vi "CRYStatistics Editor.vi"() -> ()   [LabVIEW 2013]
uses:
  <vilib>/Utility/miscctls.llb/LVBoundsTypeDef.ctl
  Typedef Control/CRYStatistic cluster.ctl
  CRYProject/CRYProject Editor Global.vi
  CRYWindow/SubVI/CRYMain Sub Window Global.vi
  CRYStepSetup/CRYStepSetup Global.vi
  CRYMainGlobal.vi
panel:
  out "Statistics Bk":T1
  in  "CurLibChange":bool caption="Add Lib"
  out "Load_State":bool
  out "EndFlag":bool
  in  "Add Lib":bool=TRUE
  in  "AddStep":bool
  in  "Board Tab":enum32{"Page 1"}(tab)
  in  "Main Tab":enum32{"Setting", "Help"}(tab)
  in  "Sel_Idx":i16
  out "No.Cur Sel":i32 caption="选择曲线个数"
  in  "Mode":u16(slide)
  in  "Sub2 Tab":enum32{"Page 1"}(tab)
  in  "Result Listbox":i32[](listbox)
  in  "AbsMar_StaDev":bool caption="绝对容限标准差"
  in  "Res sigma":i32 caption="+/- 西格玛"
  in  "Mar_Stan Dev":bool caption="容限标准差"
  in  "Margin Mean":bool caption="容限平均值"
  in  "Overall Yield":bool caption="总合格(%)"
  in  "Individual Lim":bool caption="单结果合格(%)"
  out "Result":bool caption="结果"
  in  "Sub1 Tab":enum32{"Page 1"}(tab)
  in  "Data Listbox":i32[](listbox)
  in  "No.Ranked(BF)":i32=1 caption="排" min=1 step=1
  out "LSL Unit":string
  out "USL Unit":string
  in  "LSL":dbl format="%#.2p"
  in  "USL":dbl format="%#.2p"
  in  "Worst Fit":bool caption="最差适合均值"
  in  "Best Fit":bool caption="最佳适合均值"
  in  "Ppk":bool
  in  "Pp":bool
  in  "Abs Stan Dev":bool caption="绝对标准偏差"
  in  "Data sigma":i32 caption="+/- 西格玛"
  in  "Stan Dev":bool caption="标准偏差"
  in  "Mean":bool caption="平均值"
  in  "Min":bool caption="最小值"
  in  "Max":bool caption="最大值"
  out "Data":bool caption="数据"
  in  "No.Ranked(WF)":i32=1 caption="排" min=1 step=1
  in  "Mode xyz":u16(slide) scale=0.0..2.0
  in  "Work in":u16(slide) caption="Work in:"
  in  "Help":string
  in  "Load...":bool caption="Apply"
  in  "Save As...":bool caption="Apply"
  in  "Revert":bool caption="Apply"
  in  "OK":bool caption="Apply"
  in  "Cancel":bool caption="Apply"
  in  "Hardware In":string
  in  "Calibration In":string
  in  "Channel":i32=1
  out "Set up Out":string
  in  "Set up In":string
  in  "stop":bool
  in  "Load Test":bool=TRUE
  in  "Statistics":T1
  out "VIMiniumBound":T2
  in  "Proper VI No":i32
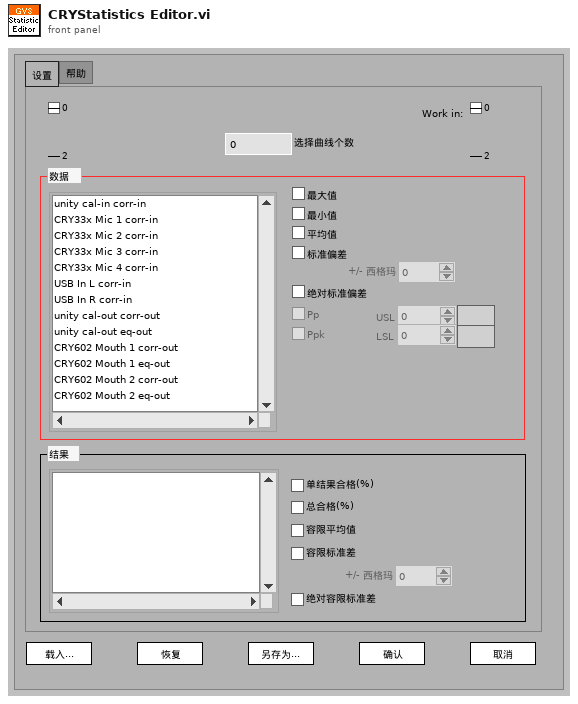
[diagram p1: front panel]
types:
  T1 = typedef "CRYStatistic cluster.ctl" = cluster{"Mode":u16, "No.Ranked(BF)":i32, "No.Ranked(WF)":i32, "Absolute Margin Standard Deviation":bool, "+/- sigma Res":i32, "Margin Standard Deviation":bool, "Margin Mean":bool, "Overall Yield":bool, "Individual Limits Yield":bool, "LSL Unit":string, "USL Unit\n":string, "LSL":dbl, "USL":dbl, "Worst Fit to Average":bool, "Best Fit to Average":bool, "Ppk":bool, "Pp":bool, "Absolute Standard Deviation":bool, "+/- sigma Dat":i32, "Standard Deviation ":bool, "Mean":bool, "Min ":bool, "Max ":bool, "No.of Curves Selected":i32, "Curves":string[], " Results":string[], "Name":string, "Help":string, "Tab Value":enum32{"Setting", "Help"}, "Work in":u16, "Mode xyz":u16}
  T2 = typedef "LVBoundsTypeDef.ctl" = cluster{"Width":u32, "Height":u32}
  T3 = typedef "CRYStep.ctl" = cluster{"No.VI":i32, "Category":string, "StepName":string, "Seq setup flattened":string, "Comment":string, "Steps config.":bool[], "Jump config":i32[], "Start":dbl, "Increment":dbl, "Name":string, "Unit":string, "Y data":u16, "Y prefix":string, "Y dB ref":dbl, "Y unit":string, "Repeat State Array":cluster{"Start":dbl, "Increment":dbl, "Count":i32, "Num":i32}[]}
  T4 = typedef "CRYData Cluster Array.ctl" = T5[]
  T5 = typedef "CRYData Cluster.ctl" = cluster{"Name":string, "Curve":cluster{"x":dbl, "y":dbl, "z":dbl}[], "X data":u16, "Y data":u16, "Z data":u16, "X axis":u16, "Y axis":u16, "Z axis":u16, "X unit":string, "Y unit":string, "Z unit":string, "X dB ref":dbl, "Y dB ref":dbl, "Z dB ref":dbl, "single val":bool, "protected":bool, "display X":bool, "display Y":bool, "display Z":bool, "Test Info":string, "Step No.":i32, "Plot Settings":cluster{"Color":u32, "Interpolation":u8, "Point Style":u8, "Line Style":u8, "Point Color":u32, "Line Width":u8, "Bar Plot Style":u8, "Fill To":i16}, "AutoProtect":bool}
  T6 = typedef "CRYResult Cluster Array.ctl" = T7[]
  T7 = typedef "CRYResult Cluster.ctl" = cluster{"Name":string, "Margin":dbl, "unit":string, "Verdict":bool, "Limit":string, "Max/Min":string, "protected":bool, "Step No.":i32, "Test Info":string, "AutoProtect":bool}
  T8 = enum16{"OK", "Yes", "YesNo", "YesNoCancel", "ReplaceAppend"}
  T9 = enum8{"Enabled", "Disabled", "Disabled and Grayed Out"}
  T10 = cluster{"Load Test":bool, "Add Lib":bool, "OK":bool, "Cancel":bool}
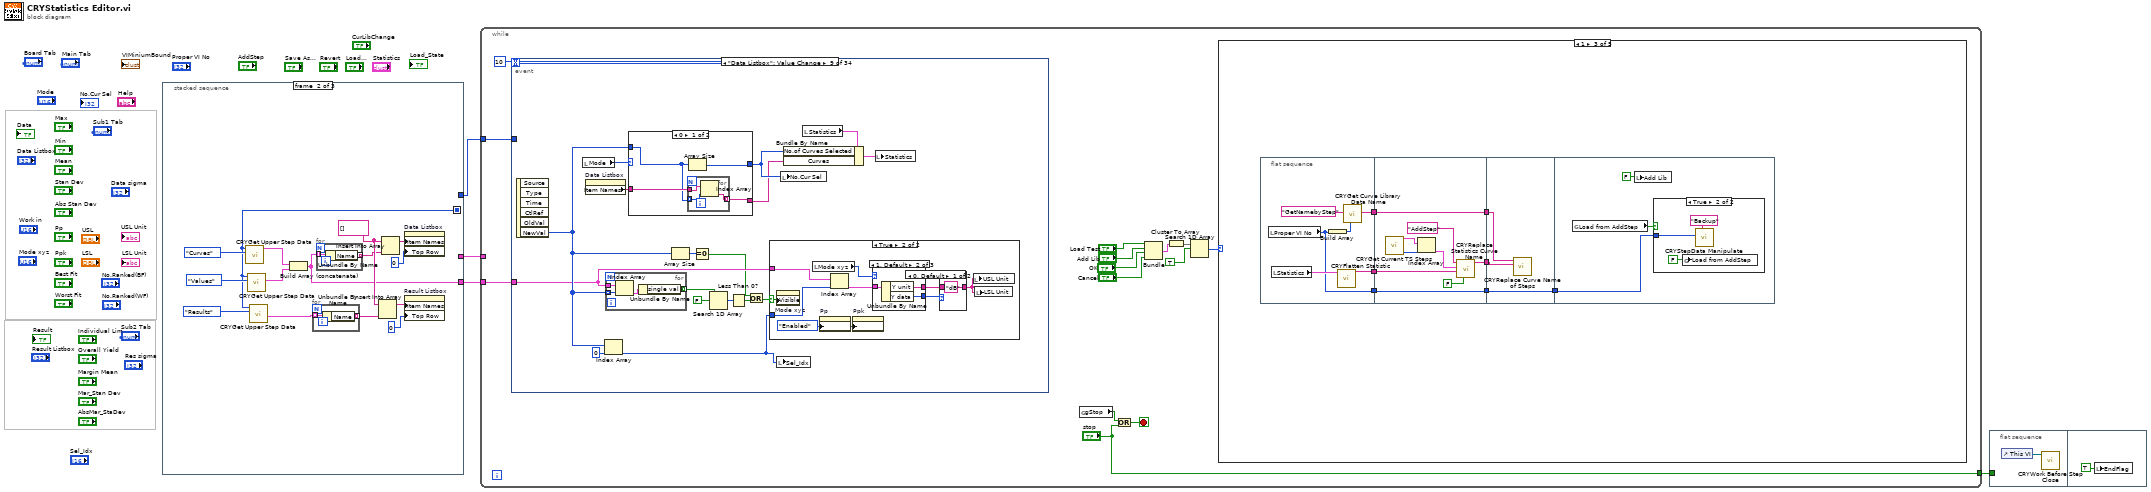
[diagram p0: block diagram]
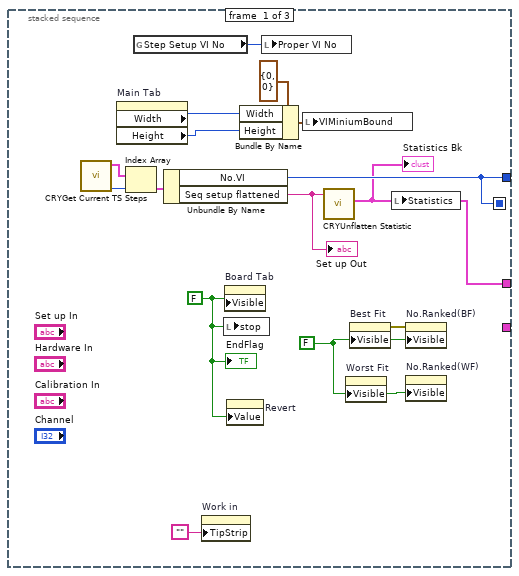
[diagram p2: hidden frame]
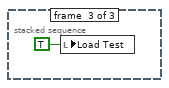
[diagram p3: hidden frame]
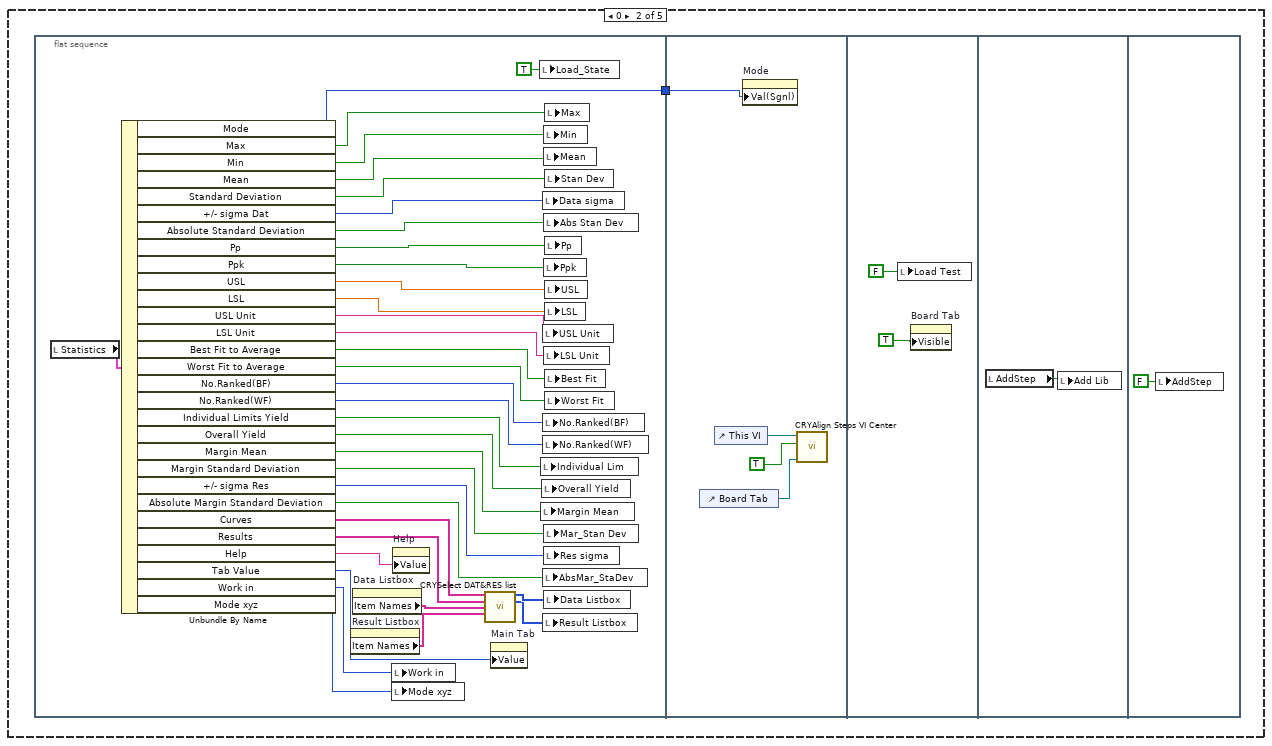
[diagram p5: hidden frame]
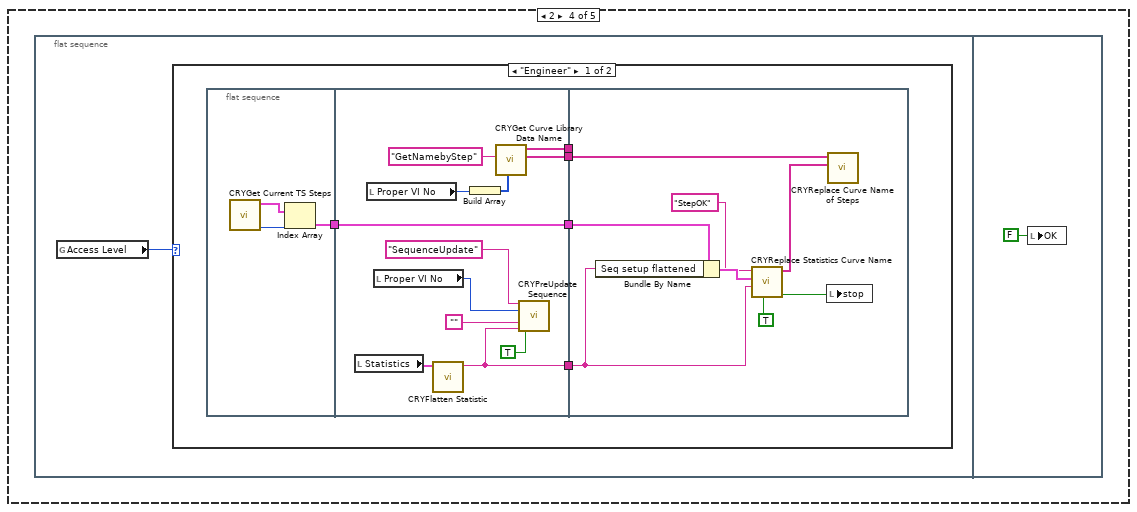
[diagram p7: hidden frame]
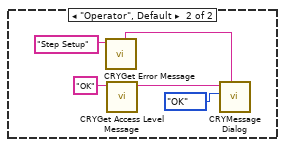
[diagram p8: hidden frame]
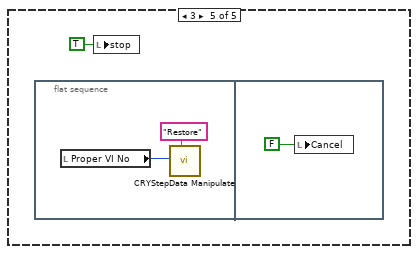
[diagram p9: hidden frame]
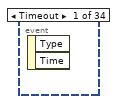
[diagram p10: hidden frame]
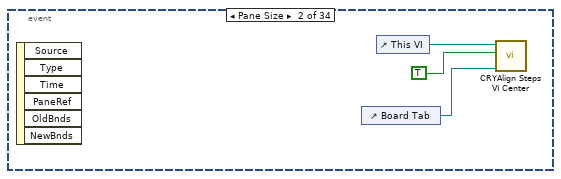
[diagram p11: hidden frame]
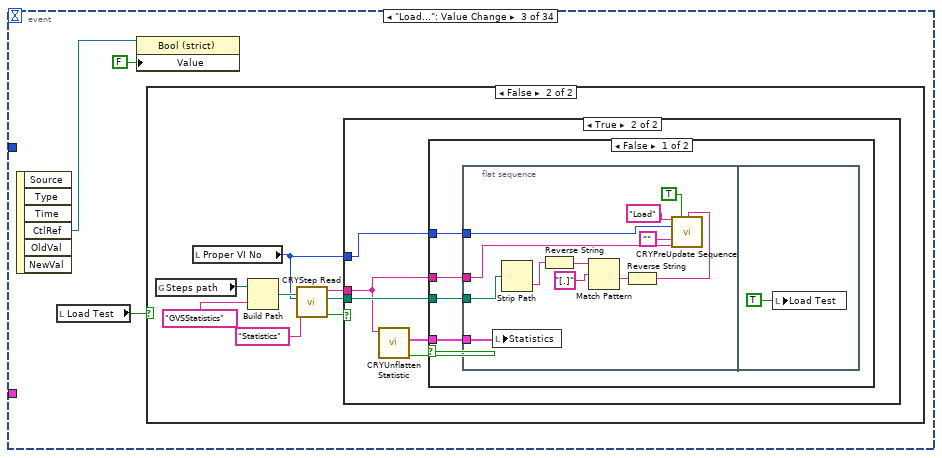
[diagram p12: hidden frame]
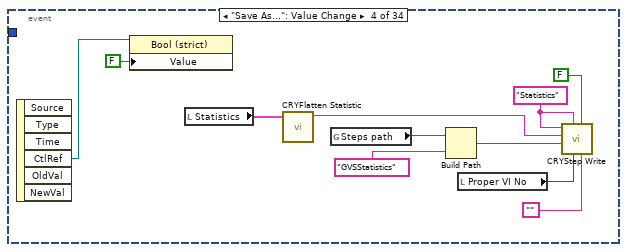
[diagram p16: hidden frame]
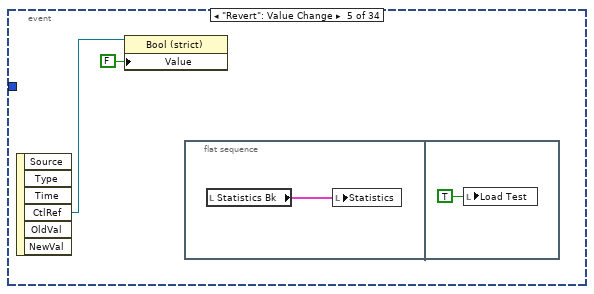
[diagram p17: hidden frame]
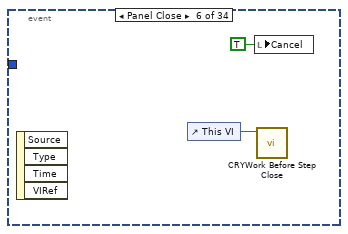
[diagram p18: hidden frame]
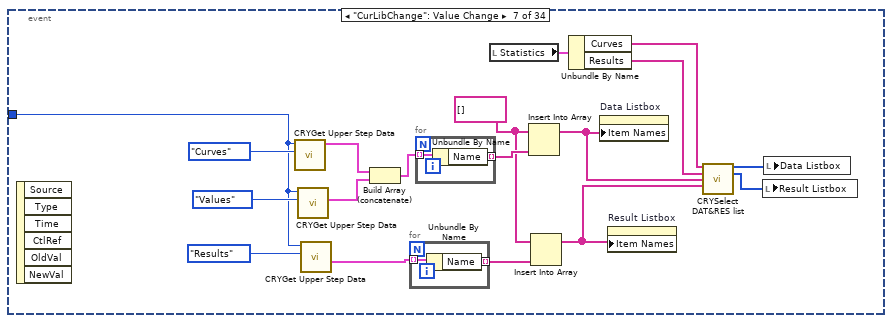
[diagram p19: hidden frame]
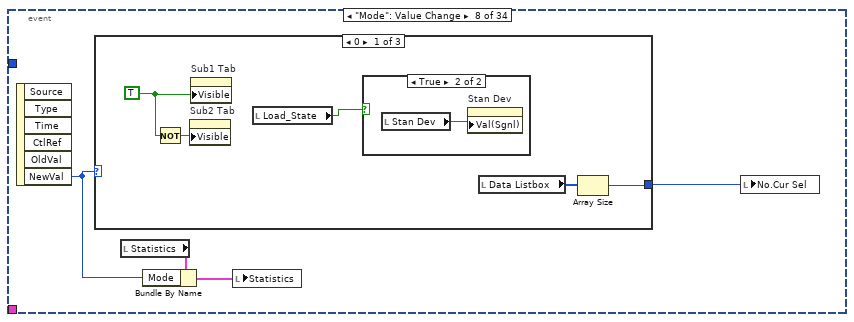
[diagram p20: hidden frame]
diagram:
  n1 = stacked-sequence {
    seq-local: [w8 _ _] -> [_ w20 _]
    tunnel: [w7 _ _] -> w4
    tunnel: [_ w23 _] -> w3
    tunnel: [w8 _ _] -> w1
    frame #0 {
      w9 = FALSE
      w6 = FALSE ("Visible")
      n2 = call "CRYGet Current TS Steps.vi"() -> ("SelectStepNumber in Tree"=w10:i32, "Steps"=w11:T3[])  [unwired: 7 in, 3 out]
      n3 = property on="Main Tab" class="TabCtl (strict)"() -> ("Width"=w16:u32, "Height"=w14:u32)  [unwired: 2 in, 2 out]
      n4 = Index Array(array=w11, index=w10) -> (element=w15:T3)
      n5 = global read "CRYProject Editor Global.vi" "Step Setup VI No"() -> (w19:i32)
      n6 = Unbundle By Name(w15) -> ("No.VI"=w8:i32, "Seq setup flattened"=w13:string)
      "Set up Out" <- w13
      n7 = property on="Work in" class="Slide (strict)"("TipStrip"="") -> ()  [unwired: 2 in, 2 out]
      n8 = local write "stop"(w6) -> ()
      n9 = property on="Board Tab" class="TabCtl (strict)"("Visible"=w6) -> ()  [unwired: 2 in, 2 out]
      n10 = property on="Revert" class="Bool (strict)"("Value"=w6) -> ()  [unwired: 2 in, 2 out]
      n11 = Bundle By Name(cluster=T2 {"Width"=0, "Height"=0} ("VIMiniumBound"), "Width"=w16, "Height"=w14) -> (w18:T2)
      n12 = local write "Proper VI No"(w19) -> ()
      n13 = local write "VIMiniumBound"(w18) -> ()
      n14 = call "CRYUnflatten Statistic.vi"("Flatten Statistics"=w13) -> ("Statistics"=w7:T1)  [unwired: 1 in, 9 out]
      "Statistics Bk" <- w7
      n15 = property on="Worst Fit" class="Bool (strict)"("Visible"=w9) -> ()  [unwired: 2 in, 2 out]
      n16 = property on="Best Fit" class="Bool (strict)"("Visible"=w9) -> (error out=w12:errorcluster)  [unwired: 2 in, 1 out]
      n17 = local write "Statistics"(w7) -> ()
      n18 = property on="No.Ranked(BF)" class="DigNum (strict)"(error in=w12, "Visible"=w9) -> ()  [unwired: 1 in, 2 out]
      n19 = property on="No.Ranked(WF)" class="DigNum (strict)"("Visible"=w9) -> ()  [unwired: 2 in, 2 out]
      "EndFlag" <- w6
    }
    frame #1 {
      w34 = string[] [] ("Item Names")
      n20 = call "CRYGet Upper Step Data.vi"("Type In"=enum16{"Curves", "Values", "Results", "WFM"}."Curves", "No.VI"=w20) -> ("Curve array"=w25:T4)  [unwired: 9 out]
      n21 = call "CRYGet Upper Step Data.vi"("Type In"=enum16{"Curves", "Values", "Results", "WFM"}."Values", "No.VI"=w20) -> ("Value array"=w24:T4)  [unwired: 9 out]
      n22 = call "CRYGet Upper Step Data.vi"("Type In"=enum16{"Curves", "Values", "Results", "WFM"}."Results", "No.VI"=w20) -> ("Result array"=w31:T6)  [unwired: 9 out]
      n23 = Build Array (concatenate)(w25, w24) -> (w23:T4)
      n24 = for {
        tunnel: w31 -> [w36] mode=indexing
        tunnel: [w35] -> w33 mode=indexing
        n25 = Unbundle By Name(w36) -> ("Name"=w35:string)
      }
      n26 = for {
        tunnel: w23 -> [w38] mode=indexing
        tunnel: [w37] -> w32 mode=indexing
        n27 = Unbundle By Name(w38) -> ("Name"=w37:string)
      }
      n28 = Insert Into Array(array=w34, new element=w33) -> (w26:string[])  [unwired: 1 in]
      n29 = Insert Into Array(array=w34, new element=w32) -> (w27:string[])  [unwired: 1 in]
      n30 = property on="Data Listbox" class="LstBox (strict)"("Item Names"=w27, "Top Row"=0) -> ()  [unwired: 2 in, 2 out]
      n31 = property on="Result Listbox" class="LstBox (strict)"("Item Names"=w26, "Top Row"=0) -> ()  [unwired: 2 in, 2 out]
    }
    frame #2 {
      n32 = local write "Load Test"(TRUE ("Load Test")) -> ()
    }
  }
  n33 = while {
    tunnel: w4 -> [_]
    tunnel: w3 -> [w45]
    tunnel: ["stop"] -> w2
    tunnel: w1 -> [w42]
    stop <- w47 stop-if-true
    n34 = event shown="[8] \"Data Listbox\": Value Change" {
      selector: _ -> [_ _ _ _ _ _ _ _ _ _ _ _ _ _ _ _ _ _ _ _ _ _ _ _ _ _ _ _ _ _ _ _ _ _]
      dyn-events: _ -> [_ _ _ _ _ _ _ _ _ _ _ _ _ _ _ _ _ _ _ _ _ _ _ _ _ _ _ _ _ _ _ _ _ _]
      timeout: 10 -> [_ _ _ _ _ _ _ _ _ _ _ _ _ _ _ _ _ _ _ _ _ _ _ _ _ _ _ _ _ _ _ _ _ _]
      tunnel: w45 -> [_ _ _ _ _ _ _ _ w283 _ _ _ _ _ _ _ _ _ _ _ _ _ _ _ _ _ _ _ _ _ _ w455 _ _]
      tunnel: w42 -> [_ _ _ _ _ _ w221 _ _ _ _ _ _ _ _ _ _ _ _ _ _ _ _ _ _ _ _ _ _ _ _ _ _ _]
      event Timeout {
        n35 = event-data() -> ()  [unwired: 3 out]
      }
      event Pane Size {
        n36 = event-data() -> ()  [unwired: 7 out]
        n37 = control-ref of="Board Tab"() -> (w169:refnum<vi>)
        n38 = control-ref of="This VI"() -> (w168:refnum<vi>)
        n39 = call "CRYAlign Steps VI Center.vi"("Tab2"=w169, "Input/Output"=TRUE ("Preview"), "VIRef"=w168) -> ()  [unwired: 1 in, 8 out]
      }
      event "Load...": Value Change {
        n40 = event-data() -> ("CtlRef"=w171:refnum<vi>)  [unwired: 6 out]
        n41 = local read "Load Test"() -> (w173:bool)
        n42 = property class="Bool (strict)"(reference=w171, "Value"=FALSE) -> ()  [unwired: 1 in, 2 out]
        n43 = case shown="False" w173 {
          frame True {
          }
          frame False {
            n44 = global read "CRYMainGlobal.vi" "Steps path"() -> (w180:path)
            n45 = local read "Proper VI No"() -> (w175:i32)
            n46 = Build Path(base path=w180, name or relative path="GVSStatistics") -> (appended path=w179:path)
            n47 = call "CRYStep Read.vi"("Category Name"="Statistics", "Proper VI No"=w175, "Step File Path"=w179) -> ("status"=w177:bool, "selected path"=w174:path, "Flatten Step"=w176:string)  [unwired: 1 in, 3 out]
            n48 = case shown="True" w177 {
              tunnel: w176 -> [_ w182]
              tunnel: w175 -> [_ w184]
              tunnel: w174 -> [_ w183]
              frame False {
              }
              frame True {
                n49 = call "CRYUnflatten Statistic.vi"("Flatten Statistics"=w182) -> ("Error?"=w186:bool, "Statistics"=w185:T1)  [unwired: 9 out]
                n50 = case shown="False" w186 {
                  tunnel: w185 -> [w190 _]
                  tunnel: w184 -> [w189 _]
                  tunnel: w183 -> [w188 _]
                  tunnel: w182 -> [w187 _]
                  frame False {
                    n51 = flat-sequence {
                      tunnel: w190 -> [w202]
                      tunnel: w189 -> [w199]
                      tunnel: w188 -> [w198]
                      tunnel: w187 -> [w197]
                      frame #0 {
                        n52 = local write "Statistics"(w202) -> ()
                        n53 = Strip Path(path=w198) -> (name=w192:string)  [unwired: 1 out]
                        n54 = Reverse String(1:w192) -> (0:w194:string)
                        n55 = Match Pattern(string=w194, regular expression="[.]") -> (after substring=w195:string)  [unwired: 4 out]
                        n56 = Reverse String(1:w195) -> (0:w191:string)
                        n57 = call "CRYPreUpdate Sequence.vi"("EventName"="Load", "StepName Arg3"=w191, "Proper VI No"=w199, "Project View Step Name Identifier Arg1"="", "Step flattened Arg2"=w197, "AllChangeFlg"=TRUE ("Name/Identifier")) -> ()  [unwired: 10 in]
                      }
                      frame #1 {
                        n58 = local write "Load Test"(TRUE ("Load Test")) -> ()
                      }
                    }
                  }
                  frame True {
                  }
                }
              }
            }
          }
        }
      }
      event "Save As...": Value Change {
        w208 = "Statistics" ("Step File Name")
        n59 = event-data() -> ("CtlRef"=w204:refnum<vi>)  [unwired: 6 out]
        n60 = property class="Bool (strict)"(reference=w204, "Value"=FALSE) -> ()  [unwired: 1 in, 2 out]
        n61 = local read "Statistics"() -> (w207:T1)
        n62 = call "CRYFlatten Statistic.vi"("Statistics"=w207) -> ("Flatten Statistics String"=w206:string)  [unwired: 1 in, 9 out]
        n63 = global read "CRYMainGlobal.vi" "Steps path"() -> (w210:path)
        n64 = Build Path(base path=w210, name or relative path="GVSStatistics") -> (appended path=w209:path)
        n65 = local read "Proper VI No"() -> (w213:i32)
        n66 = call "CRYStep Write.vi"("StepIdentifier"="", "Default"=FALSE, "Proper VI No"=w213, "Category Name"=w208, "Step File Path"=w209, "Step flattened"=w206, "Step File Name"=w208) -> ()  [unwired: 1 in, 4 out]
      }
      event "Revert": Value Change {
        n67 = event-data() -> ("CtlRef"=w215:refnum<vi>)  [unwired: 6 out]
        n68 = property class="Bool (strict)"(reference=w215, "Value"=FALSE) -> ()  [unwired: 1 in, 2 out]
        n69 = flat-sequence {
          frame #0 {
            n70 = local read "Statistics Bk"() -> (w217:T1)
            n71 = local write "Statistics"(w217) -> ()
          }
          frame #1 {
            n72 = local write "Load Test"(TRUE ("Load Test")) -> ()
          }
        }
      }
      event Panel Close {
        n73 = event-data() -> ()  [unwired: 5 out]
        n74 = control-ref of="This VI"() -> (w220:refnum<vi>)
        n75 = local write "Cancel"(TRUE ("Cancel")) -> ()
        n76 = call "CRYWork Before Step Close.vi"("StepVI Ref"=w220) -> ()  [unwired: 11 in]
      }
      event "CurLibChange": Value Change {
        w229 = string[] [] ("Item Names")
        n77 = event-data() -> ()  [unwired: 7 out]
        n78 = call "CRYGet Upper Step Data.vi"("Type In"=enum16{"Curves", "Values", "Results", "WFM"}."Curves", "No.VI"=w221) -> ("Curve array"=w236:T4)  [unwired: 9 out]
        n79 = call "CRYGet Upper Step Data.vi"("Type In"=enum16{"Curves", "Values", "Results", "WFM"}."Values", "No.VI"=w221) -> ("Value array"=w237:T4)  [unwired: 9 out]
        n80 = call "CRYGet Upper Step Data.vi"("Type In"=enum16{"Curves", "Values", "Results", "WFM"}."Results", "No.VI"=w221) -> ("Result array"=w232:T6)  [unwired: 9 out]
        n81 = Build Array (concatenate)(w236, w237) -> (w238:T4)
        n82 = for {
          tunnel: w232 -> [w240] mode=indexing
          tunnel: [w239] -> w230 mode=indexing
          n83 = Unbundle By Name(w240) -> ("Name"=w239:string)
        }
        n84 = for {
          tunnel: w238 -> [w242] mode=indexing
          tunnel: [w241] -> w231 mode=indexing
          n85 = Unbundle By Name(w242) -> ("Name"=w241:string)
        }
        n86 = local read "Statistics"() -> (w224:T1)
        n87 = Insert Into Array(array=w229, new element=w231) -> (w226:string[])  [unwired: 1 in]
        n88 = Insert Into Array(array=w229, new element=w230) -> (w225:string[])  [unwired: 1 in]
        n89 = Unbundle By Name(w224) -> ("Curves"=w223:string[], "Results"=w222:string[])
        n90 = property on="Data Listbox" class="LstBox (strict)"("Item Names"=w226) -> ()  [unwired: 2 in, 2 out]
        n91 = property on="Result Listbox" class="LstBox (strict)"("Item Names"=w225) -> ()  [unwired: 2 in, 2 out]
        n92 = call "CRYSelect DAT&RES list.vi"("Selected Data Item"=w223, "Selected Result Item"=w222, "Data Names"=w226, "Result Names"=w225) -> ("Data Index"=w228:i32[], "Result Index"=w227:i32[])  [unwired: 1 in, 9 out]
        n93 = local write "Result Listbox"(w227) -> ()
        n94 = local write "Data Listbox"(w228) -> ()
      }
      event "Mode": Value Change {
        n95 = event-data() -> ("NewVal"=w243:u16)  [unwired: 6 out]
        n96 = case shown="0" w243 {
          tunnel: [w250 w256 w261] -> w246
          frame 0 {
            w248 = TRUE ("Visible")
            n97 = Not(x=w248) -> (.not. x?=w249:bool)
            n98 = property on="Sub2 Tab" class="TabCtl (strict)"("Visible"=w249) -> ()  [unwired: 2 in, 2 out]
            n99 = property on="Sub1 Tab" class="TabCtl (strict)"("Visible"=w248) -> ()  [unwired: 2 in, 2 out]
            n100 = local read "Load_State"() -> (w247:bool)
            n101 = case shown="True" w247 {
              frame False {
              }
              frame True {
                n102 = local read "Stan Dev"() -> (w252:bool)
                n103 = property on="Stan Dev" class="Bool (strict)"("Val(Sgnl)"=w252) -> ()  [unwired: 2 in, 2 out]
              }
            }
            n104 = local read "Data Listbox"() -> (w251:i32[])
            n105 = Array Size(array=w251) -> (size(s)=w250:i32)
          }
          frame 1 {
            w254 = TRUE ("Visible")
            n106 = Not(x=w254) -> (.not. x?=w255:bool)
            n107 = property on="Sub2 Tab" class="TabCtl (strict)"("Visible"=w254) -> ()  [unwired: 2 in, 2 out]
            n108 = property on="Sub1 Tab" class="TabCtl (strict)"("Visible"=w255) -> ()  [unwired: 2 in, 2 out]
            n109 = local read "Load_State"() -> (w253:bool)
            n110 = case shown="True" w253 {
              frame False {
              }
              frame True {
                n111 = local read "Mar_Stan Dev"() -> (w258:bool)
                n112 = property on="Mar_Stan Dev" class="Bool (strict)"("Val(Sgnl)"=w258) -> ()  [unwired: 2 in, 2 out]
              }
            }
            n113 = local read "Result Listbox"() -> (w257:i32[])
            n114 = Array Size(array=w257) -> (size(s)=w256:i32)
          }
          frame 2, Default {
            w260 = TRUE ("Visible")
            n115 = property on="Sub2 Tab" class="TabCtl (strict)"("Visible"=w260) -> ()  [unwired: 2 in, 2 out]
            n116 = property on="Sub1 Tab" class="TabCtl (strict)"("Visible"=w260) -> ()  [unwired: 2 in, 2 out]
            n117 = local read "Result Listbox"() -> (w262:i32[])
            n118 = local read "Data Listbox"() -> (w263:i32[])
            n119 = local read "Load_State"() -> (w259:bool)
            n120 = Array Size(array=w262) -> (size(s)=w265:i32)
            n121 = Array Size(array=w263) -> (size(s)=w264:i32)
            n122 = Add(x=w264, y=w265) -> (x+y=w261:i32)
            n123 = case shown="True" w259 {
              frame False {
              }
              frame True {
                n124 = local read "Mar_Stan Dev"() -> (w266:bool)
                n125 = local read "Stan Dev"() -> (w267:bool)
                n126 = property on="Stan Dev" class="Bool (strict)"("Val(Sgnl)"=w267) -> ()  [unwired: 2 in, 2 out]
                n127 = property on="Mar_Stan Dev" class="Bool (strict)"("Val(Sgnl)"=w266) -> ()  [unwired: 2 in, 2 out]
              }
            }
          }
        }
        n128 = local read "Statistics"() -> (w245:T1)
        n129 = Bundle By Name(cluster=w245, "Mode"=w243) -> (w244:T1)
        n130 = local write "Statistics"(w244) -> ()
        n131 = local write "No.Cur Sel"(w246) -> ()
      }
      event "Data Listbox": Value Change {
        n132 = event-data() -> ("NewVal"=w284:i32[])  [unwired: 6 out]
        n133 = local read "Mode"() -> (w281:u16)
        n134 = property on="Data Listbox" class="LstBox (strict)"() -> ("Item Names"=w278:string[])  [unwired: 2 in, 2 out]
        n135 = Index Array(array=w284, index=0) -> (element=w268:i32)
        n136 = for {
          tunnel: w284 -> [w311] mode=indexing
          tunnel: w283 -> [w310]
          tunnel: [w308] -> w273 mode=indexing
          n137 = Index Array(array=w310, index=w311) -> (element=w309:T5)
          n138 = Unbundle By Name(w309) -> ("single val"=w308:bool)
        }
        n139 = case shown="0" w281 {
          tunnel: [w315 w323] -> w280
          tunnel: [w313 w322] -> w279
          tunnel: w278 -> [w314 w320]
          tunnel: w284 -> [w312 w319]
          frame 0 {
            n140 = for {
              tunnel: w312 -> [w318] mode=indexing
              tunnel: [w316] -> w313 mode=indexing
              tunnel: w314 -> [w317]
              n141 = Index Array(array=w317, index=w318) -> (element=w316:string)
            }
            n142 = Array Size(array=w312) -> (size(s)=w315:i32)
          }
          frame 2, Default {
            n143 = local read "Result Listbox"() -> (w321:i32[])
            n144 = for {
              tunnel: w319 -> [w328] mode=indexing
              tunnel: [w326] -> w322 mode=indexing
              tunnel: w320 -> [w327]
              n145 = Index Array(array=w327, index=w328) -> (element=w326:string)
            }
            n146 = Array Size(array=w319) -> (size(s)=w325:i32)
            n147 = Array Size(array=w321) -> (size(s)=w324:i32)
            n148 = Add(x=w325, y=w324) -> (x+y=w323:i32)
          }
        }
        n149 = Array Size(array=w284) -> (size(s)=w277:i32)
        n150 = Equal To 0?(x=w277) -> (x = 0?=w275:bool)
        n151 = Search 1D Array(1D array=w273, element=FALSE) -> (index of element=w269:i32)  [unwired: 1 out]
        n152 = Less Than 0?(x=w269) -> (x < 0?=w270:bool)
        n153 = Or(x=w275, y=w270) -> (x .or. y?=w274:bool)
        n154 = case shown="True" w274 {
          selector: w274 -> [w287 w291]
          tunnel: w268 -> [_ w292]
          tunnel: w283 -> [_ w289]
          frame False {
            w285 = T9."Disabled and Grayed Out" ("Disabled")
            w286 = ""
            n155 = property on="Mode xyz" class="Slide (strict)"("Visible"=w287) -> ()  [unwired: 2 in, 2 out]
            n156 = property on="Pp" class="Bool (strict)"("DisabledEnum"=w285) -> ()  [unwired: 2 in, 2 out]
            n157 = property on="Ppk" class="Bool (strict)"("DisabledEnum"=w285) -> ()  [unwired: 2 in, 2 out]
            n158 = local write "USL Unit"(w286) -> ()
            n159 = local write "LSL Unit"(w286) -> ()
          }
          frame True {
            w288 = T9."Enabled" ("Disabled")
            n160 = property on="Mode xyz" class="Slide (strict)"("Visible"=w291) -> ()  [unwired: 2 in, 2 out]
            n161 = local read "Mode xyz"() -> (w290:u16)
            n162 = property on="Pp" class="Bool (strict)"("DisabledEnum"=w288) -> ()  [unwired: 2 in, 2 out]
            n163 = Index Array(array=w289, index=w292) -> (element=w296:T5)
            n164 = property on="Ppk" class="Bool (strict)"("DisabledEnum"=w288) -> ()  [unwired: 2 in, 2 out]
            n165 = case shown="1, Default" w290 {
              tunnel: w296 -> [w299 w302 w305]
              tunnel: [w297 w301 w304] -> w295
              tunnel: [w298 w300 w303] -> w294
              frame 0 {
                n166 = Unbundle By Name(w299) -> ("X unit"=w298:string, "X data"=w297:u16)
              }
              frame 1, Default {
                n167 = Unbundle By Name(w302) -> ("Y unit"=w300:string, "Y data"=w301:u16)
              }
              frame 2 {
                n168 = Unbundle By Name(w305) -> ("Z unit"=w303:string, "Z data"=w304:u16)
              }
            }
            n169 = case shown="0, Default" w295 {
              tunnel: w294 -> [_ w307]
              tunnel: ["dB" ("Y unit") w307] -> w293
              frame 0, Default {
              }
              frame 1 {
              }
            }
            n170 = local write "USL Unit"(w293) -> ()
            n171 = local write "LSL Unit"(w293) -> ()
          }
        }
        n172 = local write "Sel_Idx"(w268) -> ()
        n173 = local write "No.Cur Sel"(w280) -> ()
        n174 = local read "Statistics"() -> (w282:T1)
        n175 = Bundle By Name(cluster=w282, "No.of Curves Selected"=w280, "Curves"=w279) -> (w271:T1)
        n176 = local write "Statistics"(w271) -> ()
      }
      event "Result Listbox": Value Change {
        n177 = event-data() -> ("NewVal"=w335:i32[])  [unwired: 6 out]
        n178 = property on="Result Listbox" class="LstBox (strict)"() -> ("Item Names"=w330:string[])  [unwired: 2 in, 2 out]
        n179 = local read "Mode"() -> (w334:u16)
        n180 = case shown="1" w334 {
          tunnel: [w339 w347] -> w332
          tunnel: [w338 w346] -> w331
          tunnel: w330 -> [w337 w344]
          tunnel: w335 -> [w336 w343]
          frame 1 {
            n181 = for {
              tunnel: w336 -> [w342] mode=indexing
              tunnel: [w340] -> w338 mode=indexing
              tunnel: w337 -> [w341]
              n182 = Index Array(array=w341, index=w342) -> (element=w340:string)
            }
            n183 = Array Size(array=w336) -> (size(s)=w339:i32)
          }
          frame 2, Default {
            n184 = local read "Data Listbox"() -> (w345:i32[])
            n185 = for {
              tunnel: w343 -> [w352] mode=indexing
              tunnel: [w350] -> w346 mode=indexing
              tunnel: w344 -> [w351]
              n186 = Index Array(array=w351, index=w352) -> (element=w350:string)
            }
            n187 = Array Size(array=w343) -> (size(s)=w349:i32)
            n188 = Array Size(array=w345) -> (size(s)=w348:i32)
            n189 = Add(x=w349, y=w348) -> (x+y=w347:i32)
          }
        }
        n190 = local write "No.Cur Sel"(w332) -> ()
        n191 = local read "Statistics"() -> (w333:T1)
        n192 = Bundle By Name(cluster=w333, "No.of Curves Selected"=w332, "Results"=w331) -> (w329:T1)
        n193 = local write "Statistics"(w329) -> ()
      }
      event "Max": Value Change {
        n194 = event-data() -> ("NewVal"=w355:bool)  [unwired: 6 out]
        n195 = local read "Statistics"() -> (w354:T1)
        n196 = Bundle By Name(cluster=w354, "Max"=w355) -> (w353:T1)
        n197 = local write "Statistics"(w353) -> ()
      }
      event "Min": Value Change {
        n198 = event-data() -> ("NewVal"=w358:bool)  [unwired: 6 out]
        n199 = local read "Statistics"() -> (w357:T1)
        n200 = Bundle By Name(cluster=w357, "Min"=w358) -> (w356:T1)
        n201 = local write "Statistics"(w356) -> ()
      }
      event "Mean": Value Change {
        n202 = event-data() -> ("NewVal"=w361:bool)  [unwired: 6 out]
        n203 = local read "Statistics"() -> (w360:T1)
        n204 = Bundle By Name(cluster=w360, "Mean"=w361) -> (w359:T1)
        n205 = local write "Statistics"(w359) -> ()
      }
      event "Stan Dev": Value Change {
        n206 = event-data() -> ("NewVal"=w363:bool)  [unwired: 6 out]
        n207 = local read "Statistics"() -> (w365:T1)
        n208 = Bundle By Name(cluster=w365, "Standard Deviation"=w363) -> (w364:T1)
        n209 = Select(t=u8 0 ("Disabled"), s=w363, f=u8 2 ("Disabled")) -> (s? t:f=w366:u8)
        n210 = property on="Data sigma" class="DigNum (strict)"("Disabled"=w366) -> ()  [unwired: 2 in, 2 out]
        n211 = local write "Statistics"(w364) -> ()
        n212 = local read "Load_State"() -> (w362:bool)
        n213 = case shown="True" w362 {
          frame False {
          }
          frame True {
            n214 = local read "Data Listbox"() -> (w369:i32[])
            n215 = local read "Pp"() -> (w370:bool)
            n216 = property on="Pp" class="Bool (strict)"("Val(Sgnl)"=w370) -> ()  [unwired: 2 in, 2 out]
            n217 = property on="Data Listbox" class="LstBox (strict)"("Val(Sgnl)"=w369) -> ()  [unwired: 2 in, 2 out]
          }
        }
      }
      event "Data sigma": Value Change {
        n218 = event-data() -> ("NewVal"=w373:i32)  [unwired: 6 out]
        n219 = local read "Statistics"() -> (w372:T1)
        n220 = Bundle By Name(cluster=w372, "+/- sigma Dat"=w373) -> (w371:T1)
        n221 = local write "Statistics"(w371) -> ()
      }
      event "Abs Stan Dev": Value Change {
        n222 = event-data() -> ("NewVal"=w376:bool)  [unwired: 6 out]
        n223 = local read "Statistics"() -> (w375:T1)
        n224 = Bundle By Name(cluster=w375, "Absolute Standard Deviation"=w376) -> (w374:T1)
        n225 = local write "Statistics"(w374) -> ()
      }
      event "Pp": Value Change {
        n226 = event-data() -> ("NewVal"=w377:bool)  [unwired: 6 out]
        n227 = local read "Ppk"() -> (w385:bool)
        n228 = local read "Statistics"() -> (w379:T1)
        n229 = Or(x=w377, y=w385) -> (x .or. y?=w384:bool)
        n230 = Bundle By Name(cluster=w379, "Pp"=w377) -> (w378:T1)
        n231 = Select(t=u8 0, s=w384, f=u8 2 ("Disabled")) -> (s? t:f=w381:u8)
        n232 = local write "Statistics"(w378) -> ()
        n233 = local read "Load_State"() -> (w380:bool)
        n234 = property class="DigNum (strict)"("Disabled"=w381) -> ()  [unwired: 2 in, 2 out]
        n235 = property on="LSL" class="DigNum (strict)"("Disabled"=w381) -> ()  [unwired: 2 in, 2 out]
        n236 = property on="USL Unit" class="Str"("Disabled"=w381) -> ()  [unwired: 2 in, 2 out]
        n237 = property on="LSL Unit" class="Str"("Disabled"=w381) -> ()  [unwired: 2 in, 2 out]
        n238 = case shown="True" w380 {
          frame False {
          }
          frame True {
            n239 = local read "Ppk"() -> (w386:bool)
            n240 = property on="Ppk" class="Bool (strict)"("Val(Sgnl)"=w386) -> ()  [unwired: 2 in, 2 out]
          }
        }
      }
      event "Ppk": Value Change {
        n241 = event-data() -> ("NewVal"=w387:bool)  [unwired: 6 out]
        n242 = stacked-sequence {
          tunnel: w387 -> [w389]
          frame #0 {
            n243 = local read "Pp"() -> (w392:bool)
            n244 = local read "Statistics"() -> (w391:T1)
            n245 = Bundle By Name(cluster=w391, "Ppk"=w389) -> (w390:T1)
            n246 = Or(x=w389, y=w392) -> (x .or. y?=w394:bool)
            n247 = Select(t=u8 0, s=w394, f=u8 2 ("Disabled")) -> (s? t:f=w393:u8)
            n248 = local write "Statistics"(w390) -> ()
            n249 = property on="USL" class="DigNum (strict)"("Disabled"=w393) -> ()  [unwired: 2 in, 2 out]
            n250 = property on="LSL" class="DigNum (strict)"("Disabled"=w393) -> ()  [unwired: 2 in, 2 out]
            n251 = property on="USL Unit" class="Str"("Disabled"=w393) -> ()  [unwired: 2 in, 2 out]
            n252 = property on="LSL Unit" class="Str"("Disabled"=w393) -> ()  [unwired: 2 in, 2 out]
            n253 = local write "Load_State"(FALSE ("Load_State")) -> ()
          }
        }
      }
      event "USL": Value Change {
        n254 = event-data() -> ("NewVal"=w398:dbl)  [unwired: 6 out]
        n255 = local read "Statistics"() -> (w399:T1)
        n256 = Bundle By Name(cluster=w399, "USL"=w398) -> (w397:T1)
        n257 = local write "Statistics"(w397) -> ()
      }
      event "LSL": Value Change {
        n258 = event-data() -> ("NewVal"=w401:dbl)  [unwired: 6 out]
        n259 = local read "Statistics"() -> (w402:T1)
        n260 = Bundle By Name(cluster=w402, "LSL"=w401) -> (w400:T1)
        n261 = local write "Statistics"(w400) -> ()
      }
      event "Best Fit": Value Change {
        n262 = event-data() -> ("NewVal"=w404:bool)  [unwired: 6 out]
        n263 = Select(t=u8 0, s=w404, f=u8 2 ("Disabled")) -> (s? t:f=w403:u8)
        n264 = property on="No.Ranked(BF)" class="DigNum (strict)"("Disabled"=w403) -> ()  [unwired: 2 in, 2 out]
        n265 = local read "Worst Fit"() -> (w407:bool)
        n266 = property on="Worst Fit" class="Bool (strict)"("Val(Sgnl)"=w407) -> ()  [unwired: 2 in, 2 out]
      }
      event "No.Ranked(BF)": Value Change {
        n267 = event-data() -> ("NewVal"=w409:i32)  [unwired: 6 out]
        n268 = local read "Statistics"() -> (w410:T1)
        n269 = Bundle By Name(cluster=w410, "No.Ranked(BF)"=w409) -> (w408:T1)
        n270 = local write "Statistics"(w408) -> ()
      }
      event "Worst Fit": Value Change {
        n271 = event-data() -> ("NewVal"=w414:bool)  [unwired: 6 out]
        n272 = local read "Best Fit"() -> (w412:bool)
        n273 = Select(t=u8 0, s=w414, f=u8 2 ("Disabled")) -> (s? t:f=w413:u8)
        n274 = local read "Statistics"() -> (w417:T1)
        n275 = Bundle By Name(cluster=w417, "Worst Fit to Average"=w414, "Best Fit to Average"=w412) -> (w411:T1)
        n276 = property on="No.Ranked(WF)" class="DigNum (strict)"("Disabled"=w413) -> ()  [unwired: 2 in, 2 out]
        n277 = local write "Statistics"(w411) -> ()
      }
      event "No.Ranked(WF)": Value Change {
        n278 = event-data() -> ("NewVal"=w419:i32)  [unwired: 6 out]
        n279 = local read "Statistics"() -> (w420:T1)
        n280 = Bundle By Name(cluster=w420, "No.Ranked(WF)"=w419) -> (w418:T1)
        n281 = local write "Statistics"(w418) -> ()
      }
      event "Individual Lim": Value Change {
        n282 = event-data() -> ("NewVal"=w423:bool)  [unwired: 6 out]
        n283 = local read "Statistics"() -> (w422:T1)
        n284 = Bundle By Name(cluster=w422, "Individual Limits Yield"=w423) -> (w421:T1)
        n285 = local write "Statistics"(w421) -> ()
      }
      event "Overall Yield": Value Change {
        n286 = event-data() -> ("NewVal"=w426:bool)  [unwired: 6 out]
        n287 = local read "Statistics"() -> (w425:T1)
        n288 = Bundle By Name(cluster=w425, "Overall Yield"=w426) -> (w424:T1)
        n289 = local write "Statistics"(w424) -> ()
      }
      event "Margin Mean": Value Change {
        n290 = event-data() -> ("NewVal"=w429:bool)  [unwired: 6 out]
        n291 = local read "Statistics"() -> (w428:T1)
        n292 = Bundle By Name(cluster=w428, "Margin Mean"=w429) -> (w427:T1)
        n293 = local write "Statistics"(w427) -> ()
      }
      event "Mar_Stan Dev": Value Change {
        n294 = event-data() -> ("NewVal"=w440:bool)  [unwired: 6 out]
        n295 = Select(t=u8 0 ("Disabled"), s=w440, f=u8 2 ("Disabled")) -> (s? t:f=w436:u8)
        n296 = local read "Statistics"() -> (w439:T1)
        n297 = Bundle By Name(cluster=w439, "Margin Standard Deviation"=w440) -> (w435:T1)
        n298 = property on="Res sigma" class="DigNum (strict)"("Disabled"=w436) -> ()  [unwired: 2 in, 2 out]
        n299 = local write "Statistics"(w435) -> ()
        n300 = local read "Mode"() -> (w434:u16)
        n301 = local read "Load_State"() -> (w431:bool)
        n302 = Equal?(x=u16 1, y=w434) -> (x = y?=w432:bool)
        n303 = And(x=w432, y=w431) -> (x .and. y?=w430:bool)
        n304 = case shown="True" w430 {
          frame False {
          }
          frame True {
            n305 = local read "Result Listbox"() -> (w441:i32[])
            n306 = local write "Load_State"(FALSE ("Load_State")) -> ()
            n307 = property on="Result Listbox" class="LstBox (strict)"("Val(Sgnl)"=w441) -> ()  [unwired: 2 in, 2 out]
          }
        }
      }
      event "Res sigma": Value Change {
        n308 = event-data() -> ("NewVal"=w445:i32)  [unwired: 6 out]
        n309 = local read "Statistics"() -> (w444:T1)
        n310 = Bundle By Name(cluster=w444, "+/- sigma Res"=w445) -> (w443:T1)
        n311 = local write "Statistics"(w443) -> ()
      }
      event "AbsMar_StaDev": Value Change {
        n312 = event-data() -> ("NewVal"=w448:bool)  [unwired: 6 out]
        n313 = local read "Statistics"() -> (w447:T1)
        n314 = Bundle By Name(cluster=w447, "Absolute Margin Standard Deviation"=w448) -> (w446:T1)
        n315 = local write "Statistics"(w446) -> ()
      }
      event "Work in": Value Change {
        n316 = event-data() -> ("NewVal"=w451:u16)  [unwired: 6 out]
        n317 = local read "Statistics"() -> (w450:T1)
        n318 = Bundle By Name(cluster=w450, "Work in"=w451) -> (w449:T1)
        n319 = local write "Statistics"(w449) -> ()
      }
      event "Mode xyz": Value Change {
        n320 = event-data() -> ("NewVal"=w453:u16)  [unwired: 6 out]
        n321 = local read "Sel_Idx"() -> (w454:i16)
        n322 = Index Array(array=w455, index=w454) -> (element=w452:T5)
        n323 = local read "Statistics"() -> (w460:T1)
        n324 = Bundle By Name(cluster=w460, "Mode xyz"=w453) -> (w459:T1)
        n325 = case shown="0" w453 {
          tunnel: w452 -> [w463 w466 w469]
          tunnel: [w461 w465 w468] -> w458
          tunnel: [w462 w464 w467] -> w457
          frame 0 {
            n326 = Unbundle By Name(w463) -> ("X unit"=w462:string, "X data"=w461:u16)
          }
          frame 1, Default {
            n327 = Unbundle By Name(w466) -> ("Y unit"=w464:string, "Y data"=w465:u16)
          }
          frame 2 {
            n328 = Unbundle By Name(w469) -> ("Z unit"=w467:string, "Z data"=w468:u16)
          }
        }
        n329 = local write "Statistics"(w459) -> ()
        n330 = case shown="0, Default" w458 {
          tunnel: w457 -> [_ w471]
          tunnel: ["dB" ("Y unit") w471] -> w456
          frame 0, Default {
          }
          frame 1 {
          }
        }
        n331 = local write "USL Unit"(w456) -> ()
        n332 = local write "LSL Unit"(w456) -> ()
      }
      event "Help": Value Change {
        n333 = event-data() -> ("NewVal"=w473:string)  [unwired: 6 out]
        n334 = local read "Statistics"() -> (w474:T1)
        n335 = Bundle By Name(cluster=w474, "Help"=w473) -> (w472:T1)
        n336 = local write "Statistics"(w472) -> ()
      }
      event "Main Tab": Value Change {
        n337 = event-data() -> ("NewVal"=w476:enum32{"Setting", "Help"})  [unwired: 6 out]
        n338 = local read "Statistics"() -> (w477:T1)
        n339 = Bundle By Name(cluster=w477, "Tab Value"=w476) -> (w475:T1)
        n340 = local write "Statistics"(w475) -> ()
      }
    }
    n341 = global read "CRYMain Sub Window Global.vi" "gStop"() -> (w48:bool)
    n342 = Or(x=w48, y="stop") -> (x .or. y?=w47:bool)
    n343 = Bundle("Load Test"="Load Test", "Add Lib"="Add Lib", "OK"="OK", "Cancel"="Cancel") -> (w52:T10)  [unwired: 1 out]
    n344 = Cluster To Array(cluster=w52) -> (array=w51:bool[])
    n345 = Search 1D Array(1D array=w51, element=TRUE) -> (index of element=w49:i32)  [unwired: 1 out]
    n346 = case shown="1" w49 {
      frame Default {
      }
      frame 0 {
        n347 = flat-sequence {
          tunnel: [w59] -> w54
          tunnel: w54 -> [w90]
          frame #0 {
            n348 = local read "Statistics"() -> (w89:T1)
            n349 = Unbundle By Name(w89) -> ("Mode"=w59:u16, "Max"=w86:bool, "Min"=w85:bool, "Mean"=w84:bool, "Standard Deviation"=w69:bool, "+/- sigma Dat"=w82:i32, "Absolute Standard Deviation"=w83:bool, "Pp"=w68:bool, "Ppk"=w67:bool, "USL"=w76:dbl, "LSL"=w75:dbl, "USL Unit"=w81:string, "LSL Unit"=w80:string, "Best Fit to Average"=w66:bool, "Worst Fit to Average"=w65:bool, "No.Ranked(BF)"=w79:i32, "No.Ranked(WF)"=w78:i32, "Individual Limits Yield"=w70:bool, "Overall Yield"=w71:bool, "Margin Mean"=w72:bool, "Margin Standard Deviation"=w64:bool, "+/- sigma Res"=w77:i32, "Absolute Margin Standard Deviation"=w73:bool, "Curves"=w88:string[], "Results"=w87:string[], "Help"=w60:string, "Tab Value"=w58:enum32{"Setting", "Help"}, "Work in"=w56:u16, "Mode xyz"=w55:u16)
            n350 = property on="Result Listbox" class="LstBox (strict)"() -> ("Item Names"=w61:string[])  [unwired: 2 in, 2 out]
            n351 = property on="Data Listbox" class="LstBox (strict)"() -> ("Item Names"=w62:string[])  [unwired: 2 in, 2 out]
            n352 = local write "Work in"(w56) -> ()
            n353 = local write "Mode xyz"(w55) -> ()
            n354 = property on="Help" class="Str"("Value"=w60) -> ()  [unwired: 2 in, 2 out]
            n355 = call "CRYSelect DAT&RES list.vi"("Selected Data Item"=w88, "Selected Result Item"=w87, "Data Names"=w62, "Result Names"=w61) -> ("Data Index"=w74:i32[], "Result Index"=w63:i32[])  [unwired: 1 in, 9 out]
            n356 = property on="Main Tab" class="TabCtl (strict)"("Value"=w58) -> ()  [unwired: 2 in, 2 out]
            n357 = local write "Load_State"(TRUE ("Load_State")) -> ()
            n358 = local write "Individual Lim"(w70) -> ()
            n359 = local write "Margin Mean"(w72) -> ()
            n360 = local write "Overall Yield"(w71) -> ()
            n361 = local write "Data sigma"(w82) -> ()
            n362 = local write "USL Unit"(w81) -> ()
            n363 = local write "No.Ranked(BF)"(w79) -> ()
            n364 = local write "No.Ranked(WF)"(w78) -> ()
            n365 = local write "AbsMar_StaDev"(w73) -> ()
            n366 = local write "Result Listbox"(w63) -> ()
            n367 = local write "Min"(w85) -> ()
            n368 = local write "Mean"(w84) -> ()
            n369 = local write "Abs Stan Dev"(w83) -> ()
            n370 = local write "Ppk"(w67) -> ()
            n371 = local write "LSL Unit"(w80) -> ()
            n372 = local write "Mar_Stan Dev"(w64) -> ()
            n373 = local write "Res sigma"(w77) -> ()
            n374 = local write "Data Listbox"(w74) -> ()
            n375 = local write "Max"(w86) -> ()
            n376 = local write "Stan Dev"(w69) -> ()
            n377 = local write "Pp"(w68) -> ()
            n378 = local write "USL"(w76) -> ()
            n379 = local write "LSL"(w75) -> ()
            n380 = local write "Best Fit"(w66) -> ()
            n381 = local write "Worst Fit"(w65) -> ()
          }
          frame #1 {
            n382 = control-ref of="Board Tab"() -> (w92:refnum<vi>)
            n383 = control-ref of="This VI"() -> (w91:refnum<vi>)
            n384 = property on="Mode" class="Slide (strict)"("Val(Sgnl)"=w90) -> ()  [unwired: 2 in, 2 out]
            n385 = call "CRYAlign Steps VI Center.vi"("Tab2"=w92, "Input/Output"=TRUE ("Preview"), "VIRef"=w91) -> ()  [unwired: 1 in, 8 out]
          }
          frame #2 {
            n386 = local write "Load Test"(FALSE ("Load Test")) -> ()
            n387 = property on="Board Tab" class="TabCtl (strict)"("Visible"=TRUE) -> ()  [unwired: 2 in, 2 out]
          }
          frame #3 {
            n388 = local read "AddStep"() -> (w96:bool)
            n389 = local write "Add Lib"(w96) -> ()
          }
          frame #4 {
            n390 = local write "AddStep"(FALSE ("AddStep")) -> ()
          }
        }
      }
      frame 1 {
        n391 = flat-sequence {
          tunnel: [w107] -> w104
          tunnel: [w106] -> w103
          tunnel: [w105] -> w98
          tunnel: w104 -> [w119]
          tunnel: w103 -> [w114]
          tunnel: [w119] -> w102
          tunnel: [w113] -> w101
          tunnel: [w111] -> w99
          tunnel: w98 -> [w111]
          tunnel: w102 -> [w121]
          tunnel: w101 -> [w122]
          tunnel: [w120] -> w100
          tunnel: w99 -> [w120]
          tunnel: w100 -> [w123]
          frame #0 {
            n392 = local read "Proper VI No"() -> (w105:i32)
            n393 = local read "Statistics"() -> (w108:T1)
            n394 = Build Array(w105) -> (w110:i32[])
            n395 = call "CRYFlatten Statistic.vi"("Statistics"=w108) -> ("Flatten Statistics String"=w106:string)  [unwired: 10 in]
            n396 = call "CRYGet Curve Library Data Name.vi"("nData"=w110, "sAction"="GetNamebyStep" ("sOption")) -> ("sNames"=w107:string[])  [unwired: 6 in, 3 out]
          }
          frame #1 {
            n397 = call "CRYGet Current TS Steps.vi"() -> ("SelectStepNumber in Tree"=w116:i32, "Steps"=w117:T3[])  [unwired: 1 in, 9 out]
            n398 = Index Array(array=w117, index=w116) -> (element=w115:T3)
            n399 = call "CRYReplace Statistics Curve Name.vi"("IsMessage"=FALSE, "Step Set up In"=w114, "Setup in"=w115, "Type In"="AddStep") -> ("Inserted Names Out"=w113:string[])  [unwired: 6 in, 1 out]
          }
          frame #2 {
            n400 = call "CRYReplace Curve Name of Steps.vi"("New Name"=w122, "Old Name"=w121) -> ()  [unwired: 9 in, 1 out]
          }
          frame #3 {
            n401 = global read "CRYStepSetup Global.vi" "Load from AddStep"() -> (w124:bool)
            n402 = local write "Add Lib"(FALSE ("Add Lib")) -> ()
            n403 = case shown="True" w124 {
              tunnel: w123 -> [_ w127]
              frame False {
              }
              frame True {
                n404 = global write "CRYStepSetup Global.vi" "Load from AddStep"(FALSE ("Load from AddStep")) -> ()
                n405 = call "CRYStepData Manipulate.vi"("sAction"="Backup", "StepNo."=w127) -> ()  [unwired: 10 in]
              }
            }
          }
        }
      }
      frame 2 {
        n406 = flat-sequence {
          frame #0 {
            n407 = global read "CRYMainGlobal.vi" "Access Level"() -> (w129:enum16{"Engineer", "Technician", "Operator"})
            n408 = case shown="\"Engineer\"" w129 {
              frame "Engineer" {
                n409 = flat-sequence {
                  tunnel: [w135] -> w134
                  tunnel: w134 -> [w144]
                  tunnel: [w144] -> w133
                  tunnel: [w143] -> w132
                  tunnel: [w139] -> w131
                  tunnel: [w138] -> w130
                  tunnel: w133 -> [w157]
                  tunnel: w132 -> [w153]
                  tunnel: w131 -> [w156]
                  tunnel: w130 -> [_]
                  frame #0 {
                    n410 = call "CRYGet Current TS Steps.vi"() -> ("SelectStepNumber in Tree"=w137:i32, "Steps"=w136:T3[])  [unwired: 1 in, 9 out]
                    n411 = Index Array(array=w136, index=w137) -> (element=w135:T3)
                  }
                  frame #1 {
                    n412 = local read "Statistics"() -> (w145:T1)
                    n413 = local read "Proper VI No"() -> (w142:i32)
                    n414 = local read "Proper VI No"() -> (w147:i32)
                    n415 = call "CRYFlatten Statistic.vi"("Statistics"=w145) -> ("Flatten Statistics String"=w143:string)  [unwired: 1 in, 9 out]
                    n416 = Build Array(w142) -> (w140:i32[])
                    n417 = call "CRYGet Curve Library Data Name.vi"("nData"=w140, "sAction"="GetNamebyStep" ("sOption")) -> ("sNames"=w139:string[], "Type Out"=w138:string[])  [unwired: 6 in, 2 out]
                    n418 = call "CRYPreUpdate Sequence.vi"("EventName"="SequenceUpdate", "Proper VI No"=w147, "Project View Step Name Identifier Arg1"="", "Step flattened Arg2"=w143, "AllChangeFlg"=TRUE ("Name/Identifier")) -> ()  [unwired: 11 in]
                  }
                  frame #2 {
                    n419 = Bundle By Name(cluster=w157, "Seq setup flattened"=w153) -> (w154:T3)
                    n420 = call "CRYReplace Statistics Curve Name.vi"("IsMessage"=TRUE, "Step Set up In"=w153, "Setup in"=w154, "Type In"="StepOK") -> ("RunFlag"=w150:bool, "Inserted Names Out"=w155:string[])  [unwired: 6 in]
                    n421 = local write "stop"(w150) -> ()
                    n422 = call "CRYReplace Curve Name of Steps.vi"("New Name"=w155, "Old Name"=w156) -> ()  [unwired: 9 in, 1 out]
                  }
                }
              }
              frame "Operator", Default {
                n423 = call "CRYGet Error Message.vi"("Kind"="Step Setup") -> ("Window Title"=w160:string)  [unwired: 5 in, 5 out]
                n424 = call "CRYGet Access Level Message.vi"("sAction"="OK") -> ("Multibyte string"=w162:string)  [unwired: 10 in]
                n425 = call "CRYMessage Dialog.vi"("Window Title"=w160, "YesNoCancel"=T8."OK", "Message Content"=w162) -> ()  [unwired: 7 in, 2 out]
              }
            }
          }
          frame #1 {
            n426 = local write "OK"(FALSE ("OK")) -> ()
          }
        }
      }
      frame 3 {
        n427 = flat-sequence {
          frame #0 {
            n428 = local read "Proper VI No"() -> (w165:i32)
            n429 = call "CRYStepData Manipulate.vi"("sAction"="Restore", "StepNo."=w165) -> ()  [unwired: 10 in]
          }
          frame #1 {
            n430 = local write "Cancel"(FALSE ("OK")) -> ()
          }
        }
        n431 = local write "stop"(TRUE ("stop")) -> ()
      }
    }
  }
  n432 = flat-sequence {
    tunnel: w2 -> [_]
    frame #0 {
      n433 = control-ref of="This VI"() -> (w478:refnum<vi>)
      n434 = call "CRYWork Before Step Close.vi"("StepVI Ref"=w478) -> ()  [unwired: 11 in]
    }
    frame #1 {
      n435 = local write "EndFlag"(TRUE ("EndFlag")) -> ()
    }
  }
